vi "Stop Core.vi"(10 "final error code":i32, 11 "Motor in":refnum<class "Motor.lvclass">) -> (3 "Motor out":refnum<class "Motor.lvclass">)   [LabVIEW 2026, in "Motor.lvlib" / "Motor.lvclass"]
doc: "<p>(<strong>Filename</strong>: <span class=\"dnl\">Actor Framework.lvlib:Actor.lvclass:Stop Core.vi</span>)</p>\n<p>Defines what the actor does before it stops. Use the <strong>final error code</strong> input to determine whether the actor shut down in response to an error.</p>\n<p>By default, this method passes the Stop message along to all <a href=\"nihelplauncher://docs/csh?context=lvcore_lvcomm_af_launch_nested_actor\">auto-stop nested actors</a>. A descendant class may override this method to define additional behavior, such as shutting down any processes the actor initiated in its override of the <a href=\"nihelplauncher://docs/csh?context=lvcore_lvcomm_af_actor_core\">Actor Core</a> method.</p>"
uses:
  Motor.lvclass
  <vilib>/ActorFramework/Actor/Actor.lvclass
  Motor.lvclass/Motor.ctl
  CTI-Grove/Examples/Sourcecode/cti-drivers-lv-visa-simple/Examples/Driver/CTIPicoVISA.lvlib
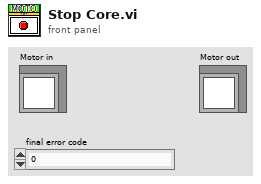
[diagram p1: front panel]
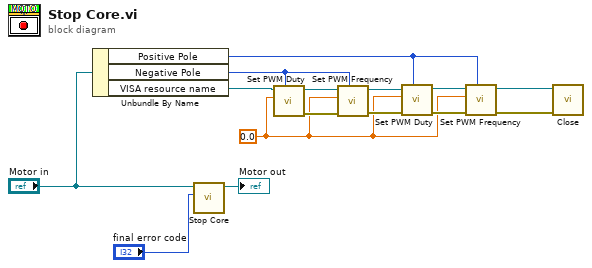
[diagram p0: block diagram]
diagram:
  w5 = sgl 0.0 ("Duty % (0-1)")
  n1 = Unbundle By Name("Motor in") -> ("Positive Pole"=w1:i32, "Negative Pole"=w2:i32, "VISA resource name"=w3:refnum<visa-resource-name>)
  n2 = call-parent "Stop Core.vi"("final error code"="final error code", "Actor in"="Motor in") -> ("Actor out"=→"Motor out":refnum<class "Motor.lvclass">)  [unwired: 9 in]
  n3 = call "Set PWM Duty.vi"("GPIO"=w2, "Duty % (0-1)"=w5, "VISA resource name in"=w3) -> ("error out"=w13:errorcluster, "VISA resource name"=w12:refnum<visa-resource-name>)  [unwired: 7 in]
  n4 = call "Set PWM Frequency.vi"("GPIO"=w2, "error in (no error)"=w13, "Freq Hz"=w5, "VISA resource name in"=w12) -> ("error out"=w11:errorcluster, "VISA resource name"=w9:refnum<visa-resource-name>)  [unwired: 6 in]
  n5 = call "Set PWM Duty.vi"("GPIO"=w1, "error in (no error)"=w11, "Duty % (0-1)"=w5, "VISA resource name in"=w9) -> ("error out"=w10:errorcluster, "VISA resource name"=w7:refnum<visa-resource-name>)  [unwired: 6 in]
  n6 = call "Set PWM Frequency.vi"("GPIO"=w1, "error in (no error)"=w10, "Freq Hz"=w5, "VISA resource name in"=w7) -> ("error out"=w8:errorcluster, "VISA resource name"=w6:refnum<visa-resource-name>)  [unwired: 6 in]
  n7 = call "Close.vi"("error in (no error)"=w8, "VISA resource name in"=w6) -> ()  [unwired: 9 in, 1 out]
